vi "shiftreg.vi"() -> ()   [LabVIEW 2022 SP3]
panel:
  out "Table":string[][](table)
  in  "stop":bool
  out "X(i-3)":dbl
  out "X(i-2)":dbl
  out "X(i-1)":dbl
  out "X(i)":u32
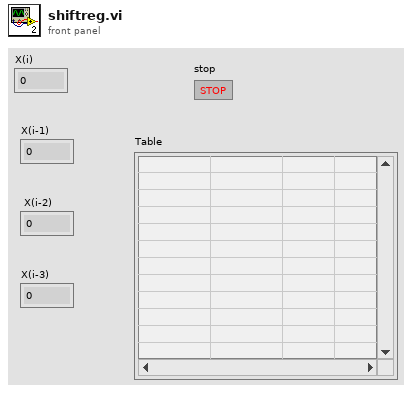
[diagram p1: front panel]
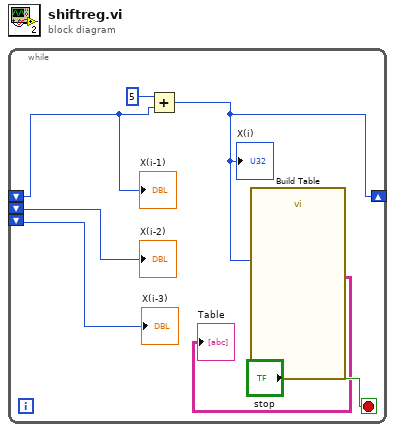
[diagram p0: block diagram]
diagram:
  n1 = while {
    shift-right: [w1] -> _
    shift-left: _ -> [w3]
    shift-left: _ -> [w5]
    shift-left: _ -> [w4]
    stop <- "stop" stop-if-true
    n2 = Add(x=5, y=w3) -> (x+y=w1:i32)
    "X(i)" <- w1
    n3 = call "Build Table"("Signals"=w1) -> ("Table"=→"Table":string[][])  [unwired: 4 in, 6 out]
    "X(i-1)" <- w3
    "X(i-2)" <- w5
    "X(i-3)" <- w4
  }
